vi "Simple_Lookup_B_tl.vi"(0 "Search String":string, 1 "Search Offset (0)":i32 min=0, 2 "Lookup Table":string[][](table), 4 "Output Offset (1)":i32=1 step=1) -> (5 "Output String":string, 6 "Output row":string[](array[string]))   [LabVIEW 2010]
doc: "Looks down the column of Lookup Table specified by Search Offset, searching for Search String. When found, outputs the string on the same row, in the column specified by Output Offset."
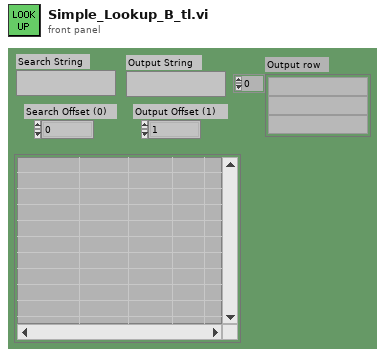
[diagram p1: front panel]
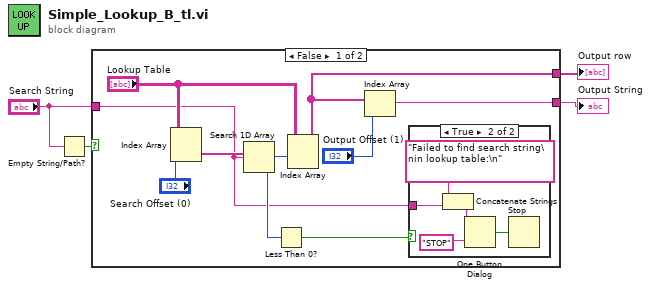
[diagram p0: block diagram]
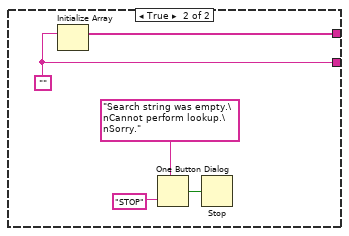
[diagram p3: hidden frame]
diagram:
  n1 = Empty String/Path?(string/path="Search String") -> (empty?=w1:bool)
  n2 = case shown="False" w1 {
    tunnel: "Search String" -> [w5 _]
    tunnel: [w9 w22] -> w3
    tunnel: [w8 w23] -> w2
    frame False {
      n3 = Index Array(array="Lookup Table", index (col)="Search Offset (0)") -> (element=w7:string[])  [unwired: 1 in]
      n4 = Search 1D Array(1D array=w7, element=w5) -> (index of element=w13:i32)  [unwired: 1 in]
      n5 = Less Than 0?(x=w13) -> (x < 0?=w6:bool)
      n6 = Index Array(array="Lookup Table", index (row)=w13) -> (element=w8:string[])  [unwired: 1 in]
      n7 = Index Array(array=w8, index="Output Offset (1)") -> (element=w9:string)
      n8 = case shown="True" w6 {
        tunnel: w5 -> [_ w14]
        frame False {
        }
        frame True {
          n9 = Concatenate Strings("Failed to find search string\nin lookup table:\n", w14) -> (w15:string)
          n10 = One Button Dialog(message=w15, button name ("OK")="STOP") -> (true=w17:bool)
          n11 = Stop(stop? (T)=w17) -> ()
        }
      }
    }
    frame True {
      w22 = ""
      n12 = Initialize Array(w22) -> (w23:string[])  [unwired: 1 in]
      n13 = One Button Dialog(message="Search string was empty.\nCannot perform lookup.\nSorry.", button name ("OK")="STOP") -> (true=w20:bool)
      n14 = Stop(stop? (T)=w20) -> ()
    }
  }
  "Output String" <- w3
  "Output row" <- w2
